vi "Get Label Properties.vi"(8 "error in":errorcluster, 11 "label ref in":T2 format="%.0x") -> (0 "error out":errorcluster, 2 "label properties":T1, 3 "label ref out":T2 format="%.0x")   [LabVIEW 2020, in "Ballard ARINC 429 Scripting.lvlib"]
uses:
  Ballard ARINC 429 Scripting.lvlib
  <vilib>/NI VeriStand/Custom Device API/Custom Device Item Ref.ctl
  Shared/Label Properties.ctl
  Constants.vi
  <vilib>/NI VeriStand/Custom Device API/Get Item Property (U16).vi
  <vilib>/NI VeriStand/Custom Device API/Get Item Property (Boolean).vi
  <vilib>/NI VeriStand/Custom Device API/Custom Device API.lvlib
  <vilib>/NI VeriStand/Custom Device API/Get Item Property (U32).vi
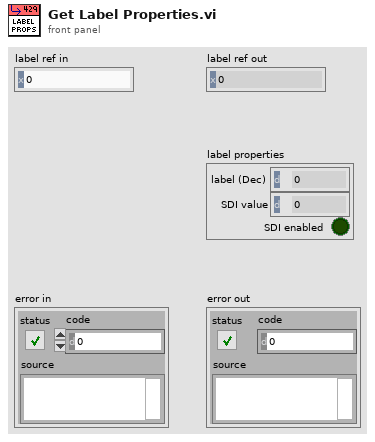
[diagram p1: front panel]
types:
  T1 = typedef "Label Properties.ctl" = cluster{"label (Dec)":u32, "SDI value":u8, "SDI enabled":bool}
  T2 = typedef "Custom Device API.lvlib/Custom Device Item Ref.ctl" = u64
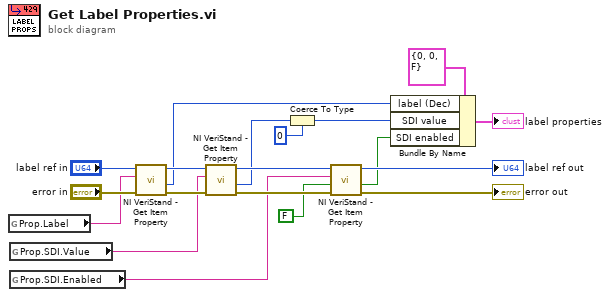
[diagram p0: block diagram]
diagram:
  n1 = global read "Constants.vi" "Prop.Label"() -> (w9:string)
  n2 = global read "Constants.vi" "Prop.SDI.Value"() -> (w8:string)
  n3 = global read "Constants.vi" "Prop.SDI.Enabled"() -> (w11:string)
  n4 = call-poly <vilib>:"NI VeriStand - Get Item Property.vi"("error in (no error)"="error in", "Property Name"=w9, "Item Ref in"="label ref in") -> ("error out"=w14:errorcluster, "Value"=w2:u32, "Item Ref out"=w15:T2)  [unwired: 5 in, 1 out]
  n5 = call-poly <vilib>:"NI VeriStand - Get Item Property.vi"("error in (no error)"=w14, "Property Name"=w8, "Item Ref in"=w15) -> ("error out"=w12:errorcluster, "Value"=w6:u16, "Item Ref out"=w13:T2)  [unwired: 5 in, 1 out]
  n6 = Coerce To Type(0:w6, 1:u8 0 ("SDI value")) -> (2:w5:u8)
  n7 = call-poly <vilib>:"NI VeriStand - Get Item Property.vi"("error in (no error)"=w12, "Default Value"=FALSE, "Property Name"=w11, "Item Ref in"=w13) -> ("error out"=→"error out":errorcluster, "Value"=w4:bool, "Item Ref out"=→"label ref out":T2)  [unwired: 4 in, 1 out]
  n8 = Bundle By Name(cluster=T1 {"label (Dec)"=0, "SDI value"=0, "SDI enabled"=FALSE} ("label properties"), "label (Dec)"=w2, "SDI value"=w5, "SDI enabled"=w4) -> (→"label properties":T1)
